vi "Field Update Sequence Field.vi"(8 "error in (no error)":errorcluster, 10 "Original Sequence Field Record":T1={"ixField"=0, "iSequenceOrder"=0, "sxFieldId"="", "sxSequenceId"="", "sDisplayName"="", "sValue"="", "sUnits"="", "nDataType"=enum."timestamp", "nNextItem"=enum."Reset", "fSystem"=FALSE, "fSystemValue"=FALSE, "fRequired"=FALSE, "fSetAtTest"=FALSE, "fTestField"=FALSE, "fDeleted"=FALSE, "fIndexed"=FALSE, "fFreeList"=FALSE}, 11 "New Sequence Field Record":T1={"ixField"=0, "iSequenceOrder"=0, "sxFieldId"="", "sxSequenceId"="", "sDisplayName"="", "sValue"="", "sUnits"="", "nDataType"=enum."timestamp", "nNextItem"=enum."Reset", "fSystem"=FALSE, "fSystemValue"=FALSE, "fRequired"=FALSE, "fSetAtTest"=FALSE, "fTestField"=FALSE, "fDeleted"=FALSE, "fIndexed"=FALSE, "fFreeList"=FALSE}) -> (0 "error out":errorcluster, 2 "Updated Field Record":T1={"ixField"=0, "iSequenceOrder"=0, "sxFieldId"="", "sxSequenceId"="", "sDisplayName"="", "sValue"="", "sUnits"="", "nDataType"=enum."timestamp", "nNextItem"=enum."Reset", "fSystem"=FALSE, "fSystemValue"=FALSE, "fRequired"=FALSE, "fSetAtTest"=FALSE, "fTestField"=FALSE, "fDeleted"=FALSE, "fIndexed"=FALSE, "fFreeList"=FALSE})   [LabVIEW 2011]
uses:
  Field Record.ctl
  Field DataTypes.ctl
  Field NextItem.ctl
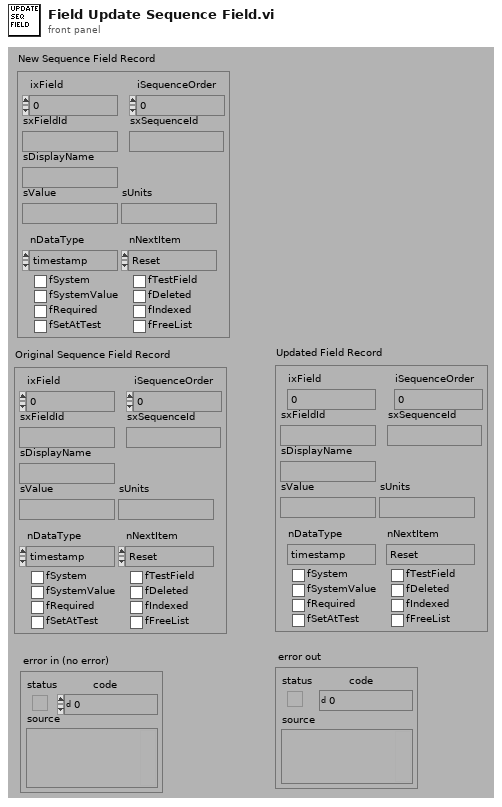
[diagram p1: front panel]
types:
  T1 = typedef "Field Record.ctl" = cluster{"ixField":i32, "iSequenceOrder":i32, "sxFieldId":string, "sxSequenceId":string, "sDisplayName":string, "sValue":string, "sUnits":string, "nDataType":T2, "nNextItem":T3, "fSystem":bool, "fSystemValue":bool, "fRequired":bool, "fSetAtTest":bool, "fTestField":bool, "fDeleted":bool, "fIndexed":bool, "fFreeList":bool}
  T2 = typedef "Field DataTypes.ctl" = enum32{"text", "numeric", "list", "timestamp", "boolean"}
  T3 = typedef "Field NextItem.ctl" = enum32{"Reset", "Retain", "Auto-Increment"}
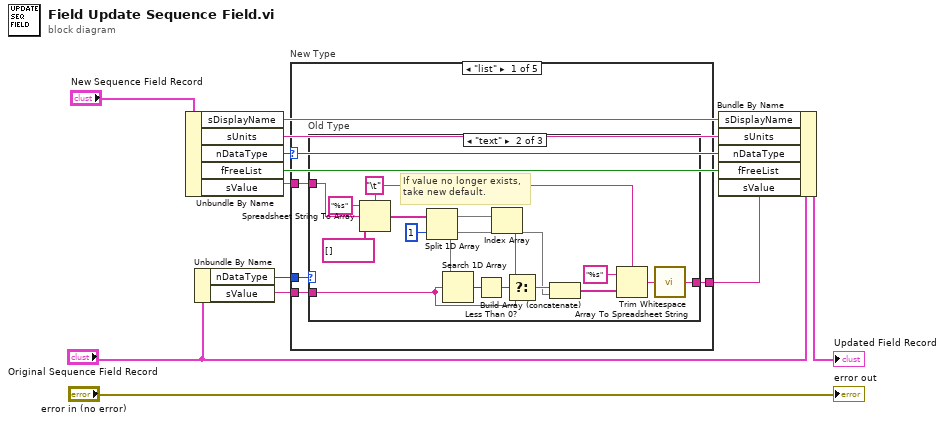
[diagram p0: block diagram]
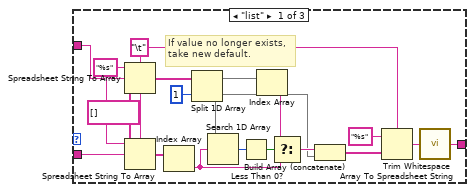
[diagram p2: hidden frame]
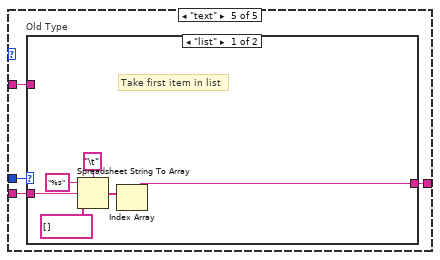
[diagram p10: hidden frame]
diagram:
  n1 = Unbundle By Name("New Sequence Field Record") -> ("sDisplayName"=w12:string, "sUnits"=w9:string, "nDataType"=w6:T2, "fFreeList"=w5:bool, "sValue"=w7:string)
  n2 = Unbundle By Name("Original Sequence Field Record") -> ("nDataType"=w8:T2, "sValue"=w10:string)
  n3 = case "New Type" shown="\"list\"" w6 {
    tunnel: [w16 w57 w63 w69 w75] -> w11
    tunnel: w10 -> [w15 w56 w62 w68 w74]
    tunnel: w7 -> [w14 w55 w61 w67 w73]
    tunnel: w8 -> [w13 w54 w60 w66 w72]
    frame "list" {
      n4 = case "Old Type" shown="\"text\"" w13 {
        tunnel: [w19 w39 w53] -> w16
        tunnel: w15 -> [w33 w37 _]
        tunnel: w14 -> [w18 w38 w53]
        frame "list" {
          w31 = string[] []
          w32 = "%s" ("format string")
          w17 = "\t" ("delimiter (Tab)")
          # "If value no longer exists,\ntake new default."
          n5 = Spreadsheet String To Array(delimiter (Tab)=w17, format string=w32, spreadsheet string=w18, array type (2D Dbl)=w31) -> (array=w28:string[])
          n6 = Spreadsheet String To Array(delimiter (Tab)=w17, format string=w32, spreadsheet string=w33, array type (2D Dbl)=w31) -> (array=w30:string[])
          n7 = Index Array(array=w30) -> (element=w29:string)  [unwired: 1 in]
          n8 = Split 1D Array(array=w28, index=1) -> (first subarray=w26:string[], second subarray=w23:string[])
          n9 = Search 1D Array(1D array=w23, element=w29) -> (index of element=w35:i32)  [unwired: 1 out]
          n10 = Less Than 0?(x=w35) -> (x < 0?=w34:bool)
          n11 = Index Array(array=w26) -> (element=w25:string)  [unwired: 1 in]
          n12 = Select(t=w25, s=w34, f=w29) -> (s? t:f=w24:string)
          n13 = Build Array (concatenate)(w24, w23) -> (w20:string[])
          n14 = Array To Spreadsheet String(delimiter (Tab)=w17, array=w20, 3:"%s" ("format string")) -> (spreadsheet string=w22:string)
          n15 = call <vilib>:"Trim Whitespace.vi"("string"=w22) -> ("trimmed string"=w19:string)  [unwired: 1 in]
        }
        frame "text" {
          w36 = "\t" ("delimiter (Tab)")
          # "If value no longer exists,\ntake new default."
          n16 = Spreadsheet String To Array(delimiter (Tab)=w36, format string="%s", spreadsheet string=w38, array type (2D Dbl)=string[] []) -> (array=w48:string[])
          n17 = Split 1D Array(array=w48, index=1) -> (first subarray=w46:string[], second subarray=w43:string[])
          n18 = Search 1D Array(1D array=w43, element=w37) -> (index of element=w52:i32)  [unwired: 1 out]
          n19 = Less Than 0?(x=w52) -> (x < 0?=w51:bool)
          n20 = Index Array(array=w46) -> (element=w45:string)  [unwired: 1 in]
          n21 = Select(t=w45, s=w51, f=w37) -> (s? t:f=w44:string)
          n22 = Build Array (concatenate)(w44, w43) -> (w40:string[])
          n23 = Array To Spreadsheet String(delimiter (Tab)=w36, array=w40, 3:"%s" ("format string")) -> (spreadsheet string=w42:string)
          n24 = call <vilib>:"Trim Whitespace.vi"("string"=w42) -> ("trimmed string"=w39:string)  [unwired: 1 in]
        }
        frame "numeric", "timestamp", "boolean" {
        }
      }
    }
    frame "numeric" {
      n25 = case "Old Type" shown="\"numeric\"" w54 {
        tunnel: [w58 w59] -> w57
        tunnel: w56 -> [w58 _]
        tunnel: w55 -> [_ w59]
        frame "numeric" {
        }
        frame "text", "list".."boolean" {
        }
      }
    }
    frame "timestamp" {
      n26 = case "Old Type" shown="\"timestamp\"" w60 {
        tunnel: [w64 w65] -> w63
        tunnel: w62 -> [w64 _]
        tunnel: w61 -> [_ w65]
        frame "timestamp" {
        }
        frame "text".."list", "boolean" {
        }
      }
    }
    frame "boolean" {
      n27 = case "Old Type" shown="\"text\"..\"timestamp\"" w66 {
        tunnel: [w70 w71] -> w69
        tunnel: w68 -> [w70 _]
        tunnel: w67 -> [_ w71]
        frame "boolean" {
        }
        frame "text".."timestamp" {
        }
      }
    }
    frame "text" {
      n28 = case "Old Type" shown="\"list\"" w72 {
        tunnel: [w76 w82] -> w75
        tunnel: w74 -> [w81 w82]
        tunnel: w73 -> [_ _]
        frame "list" {
          # "Take first item in list"
          n29 = Spreadsheet String To Array(delimiter (Tab)="\t", format string="%s", spreadsheet string=w81, array type (2D Dbl)=string[] []) -> (array=w77:string[])
          n30 = Index Array(array=w77) -> (element=w76:string)  [unwired: 1 in]
        }
        frame "text", "numeric", "timestamp", "boolean" {
        }
      }
    }
  }
  n31 = Bundle By Name(cluster="Original Sequence Field Record", "sDisplayName"=w12, "sUnits"=w9, "nDataType"=w6, "fFreeList"=w5, "sValue"=w11) -> (→"Updated Field Record":T1)
  "error out" <- "error in (no error)"
